vi "TextFile_Init.vi"(0 "object in":refnum<class "TextFile.lvclass">, 5 "error in (no error)":errorcluster) -> (14 "object out":refnum<class "TextFile.lvclass">, 19 "error out":errorcluster)   [LabVIEW 2013]
uses:
  <resource>/Framework/Providers/Symbio_GDS/ClassProviders/Provider_LvNativeClass/Templates/NativeBaseTemplate/NativeBaseTemplate.lvclass
  TextFile.lvclass
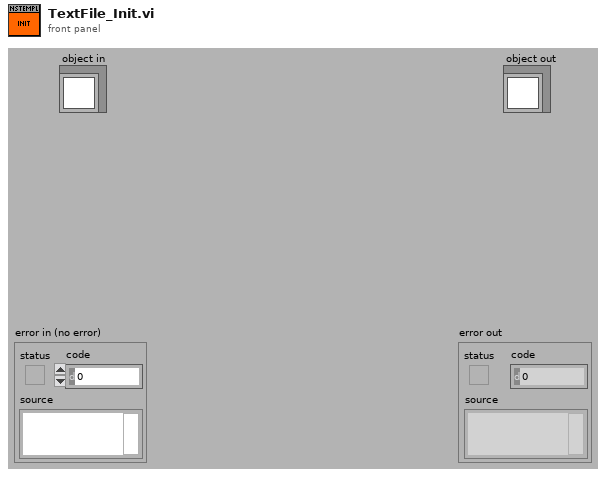
[diagram p1: front panel]
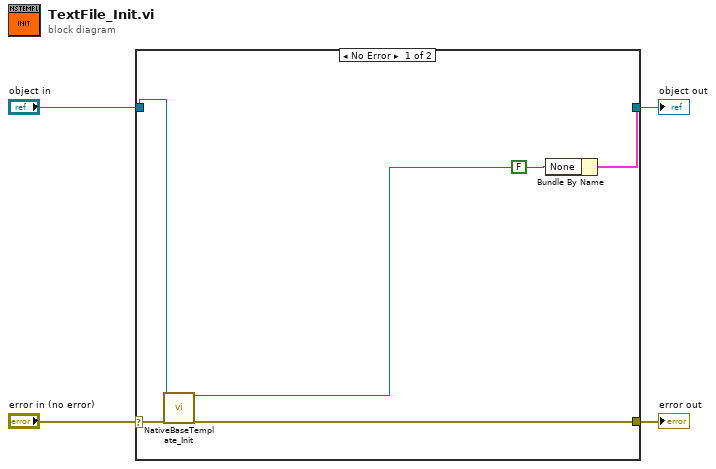
[diagram p0: block diagram]
diagram:
  n1 = case shown="No Error" "error in (no error)" {
    selector: "error in (no error)" -> [w8 w11]
    tunnel: [w10 w12] -> w4
    tunnel: "object in" -> [w6 w12]
    tunnel: [w7 w11] -> w1
    frame No Error {
      n2 = call <resource>:"NativeBaseTemplate_Init.vi"("object in"=w6, "error in (no error)"=w8) -> ("object out"=w5:refnum<class "NativeBaseTemplate.lvclass">, "error out"=w7:errorcluster)  [unwired: 16 in]
      n3 = Bundle By Name(cluster=w5, "None"=FALSE) -> (w10:cluster{})
    }
    frame Error {
    }
  }
  "object out" <- w4
  "error out" <- w1
